vi "lookupAllSettings.vi"(8 "error in (no error)":errorcluster, 9 "whichSettings":string, 11 "ICSettingsViewer in":refnum<class "ICSettingsViewer.lvclass">) -> (0 "error out":errorcluster, 3 "ICSettingsViewer out":refnum<class "ICSettingsViewer.lvclass">)   [LabVIEW 2011, in "Views.lvlib" / "Camera.lvlib" / "ICSettingsViewer.lvclass"]
uses:
  ICSettingsViewer.lvclass
  ICSettingsViewer.lvclass/ICSettingsViewer.ctl
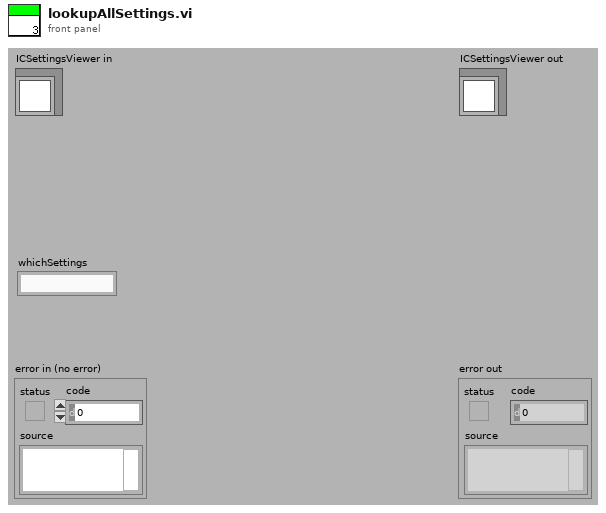
[diagram p1: front panel]
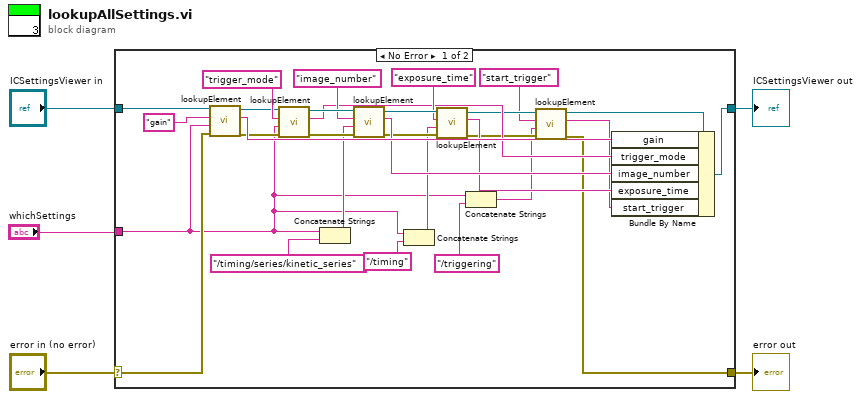
[diagram p0: block diagram]
diagram:
  n1 = case shown="No Error" "error in (no error)" {
    selector: "error in (no error)" -> [w33 w37]
    tunnel: [w13 w37] -> w4
    tunnel: [w17 w36] -> w2
    tunnel: "ICSettingsViewer in" -> [w35 w36]
    tunnel: "whichSettings" -> [w8 _]
    frame No Error {
      n2 = call "lookupElement.vi"("error in (no error)"=w33, "lookupIn"=w8, "lookupElement"="gain", "ICSettingsViewer in"=w35) -> ("error out"=w28:errorcluster, "element"=w32:string, "ICSettingsViewer out"=w30:refnum<class "ICSettingsViewer.lvclass">)  [unwired: 5 in]
      n3 = call "lookupElement.vi"("error in (no error)"=w28, "lookupIn"=w8, "lookupElement"="trigger_mode", "ICSettingsViewer in"=w30) -> ("error out"=w27:errorcluster, "element"=w16:string, "ICSettingsViewer out"=w29:refnum<class "ICSettingsViewer.lvclass">)  [unwired: 5 in]
      n4 = Concatenate Strings(w8, "/timing/series/kinetic_series") -> (w24:string)
      n5 = call "lookupElement.vi"("error in (no error)"=w27, "lookupIn"=w24, "lookupElement"="image_number", "ICSettingsViewer in"=w29) -> ("error out"=w21:errorcluster, "element"=w23:string, "ICSettingsViewer out"=w22:refnum<class "ICSettingsViewer.lvclass">)  [unwired: 5 in]
      n6 = Concatenate Strings(w8, "/timing") -> (w9:string)
      n7 = call "lookupElement.vi"("error in (no error)"=w21, "lookupIn"=w9, "lookupElement"="exposure_time", "ICSettingsViewer in"=w22) -> ("error out"=w14:errorcluster, "element"=w18:string, "ICSettingsViewer out"=w15:refnum<class "ICSettingsViewer.lvclass">)  [unwired: 5 in]
      n8 = Concatenate Strings(w8, "/triggering") -> (w6:string)
      n9 = call "lookupElement.vi"("error in (no error)"=w14, "lookupIn"=w6, "lookupElement"="start_trigger", "ICSettingsViewer in"=w15) -> ("error out"=w13:errorcluster, "element"=w11:string, "ICSettingsViewer out"=w10:refnum<class "ICSettingsViewer.lvclass">)  [unwired: 5 in]
      n10 = Bundle By Name(cluster=w10, "gain"=w32, "trigger_mode"=w16, "image_number"=w23, "exposure_time"=w18, "start_trigger"=w11) -> (w17:refnum<class "ICSettingsViewer.lvclass">)
    }
    frame Error {
    }
  }
  "error out" <- w4
  "ICSettingsViewer out" <- w2
